vi "Initialize XBOX 360 Controller.vi"(11 "XBox Device Index":i32) -> (0 "Rrror Out":errorcluster, 3 "Device ID":refnum<k1>, 5 "Joystick Info":T1(array[cluster]))   [LabVIEW 2011]
uses:
  _GlobalVariables&Libraries/ATV Program Global Variables.vi
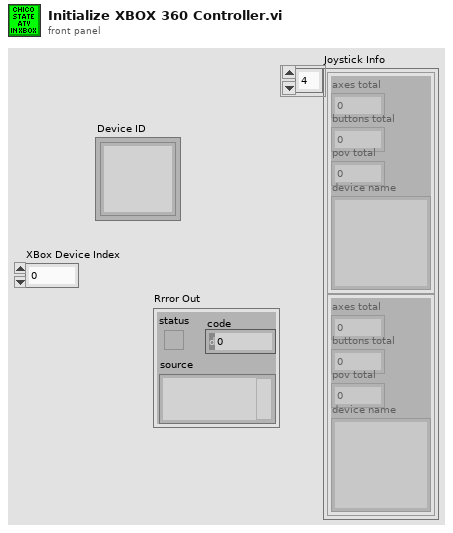
[diagram p1: front panel]
types:
  T1 = cluster{"axes total":u32, "buttons total":u32, "pov total":u32, "device name":string}[]
  T2 = cluster{"Drive Value Output String":string, "Steer Value Output String":string, "Button A":bool, "Button B":bool, "Error Out":errorcluster, "Disable XBox Drive & Steer":bool, "Disable XBox Controller":bool, "XBOX Button Trigger Time (ms)":u32, "Button X":bool, "Button Y":bool}
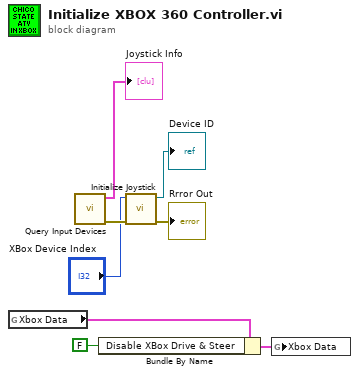
[diagram p0: block diagram]
diagram:
  n1 = global read "ATV Program Global Variables.vi" "Xbox Data"() -> (w3:T2)
  n2 = call <vilib>:"Query Input Devices.vi"() -> ("error out"=w5:errorcluster, "joystick info"=→"Joystick Info":T1)  [unwired: 8 in, 2 out]
  n3 = Bundle By Name(cluster=w3, "Disable XBox Drive & Steer"=FALSE) -> (w2:T2)
  n4 = call <vilib>:"Initialize Joystick.vi"("error in (no error)"=w5, "device index"="XBox Device Index") -> ("error out"=→"Rrror Out":errorcluster, "device ID"=→"Device ID":refnum<k1>)  [unwired: 8 in]
  n5 = global write "ATV Program Global Variables.vi" "Xbox Data"(w2) -> ()
